vi "KH TURCK ETHERNETIP RFID Read.vi"(8 "error in":errorcluster, 11 "Response Data":T2={"ItemCount"=2, "AdressItem"={"TypeID"=0, "Length"=0, "Data"={"ConnectionIdentifier"=255, "SequenceNumber"=255}}, "DataItem"={"TypeID"=178, "Length"=8, "Data"=[], "Sequence Count"=8}} {"DataItem"."Data" format="%.0x"; "DataItem"."TypeID" format="%.0x"; "AdressItem"."Data"."ConnectionIdentifier" format="%.0x"; "AdressItem"."TypeID" format="%.0x"; "ItemCount" format="%.0x"}) -> (0 "error out":errorcluster, 3 "RFID_Read":T1[](array[typedef]))   [LabVIEW 2021]
uses:
  KH TURCK ETHERNETIP TDefCluster TBEN-S2-2RFID-4DXP Input Values.ctl
  KH EthernetIP 17.19/KH_EthernetIP_Globals.vi
  KH TURCK ETHERNETIP RFID Global.vi
  KH TURCK ETHERNETIP Global.vi
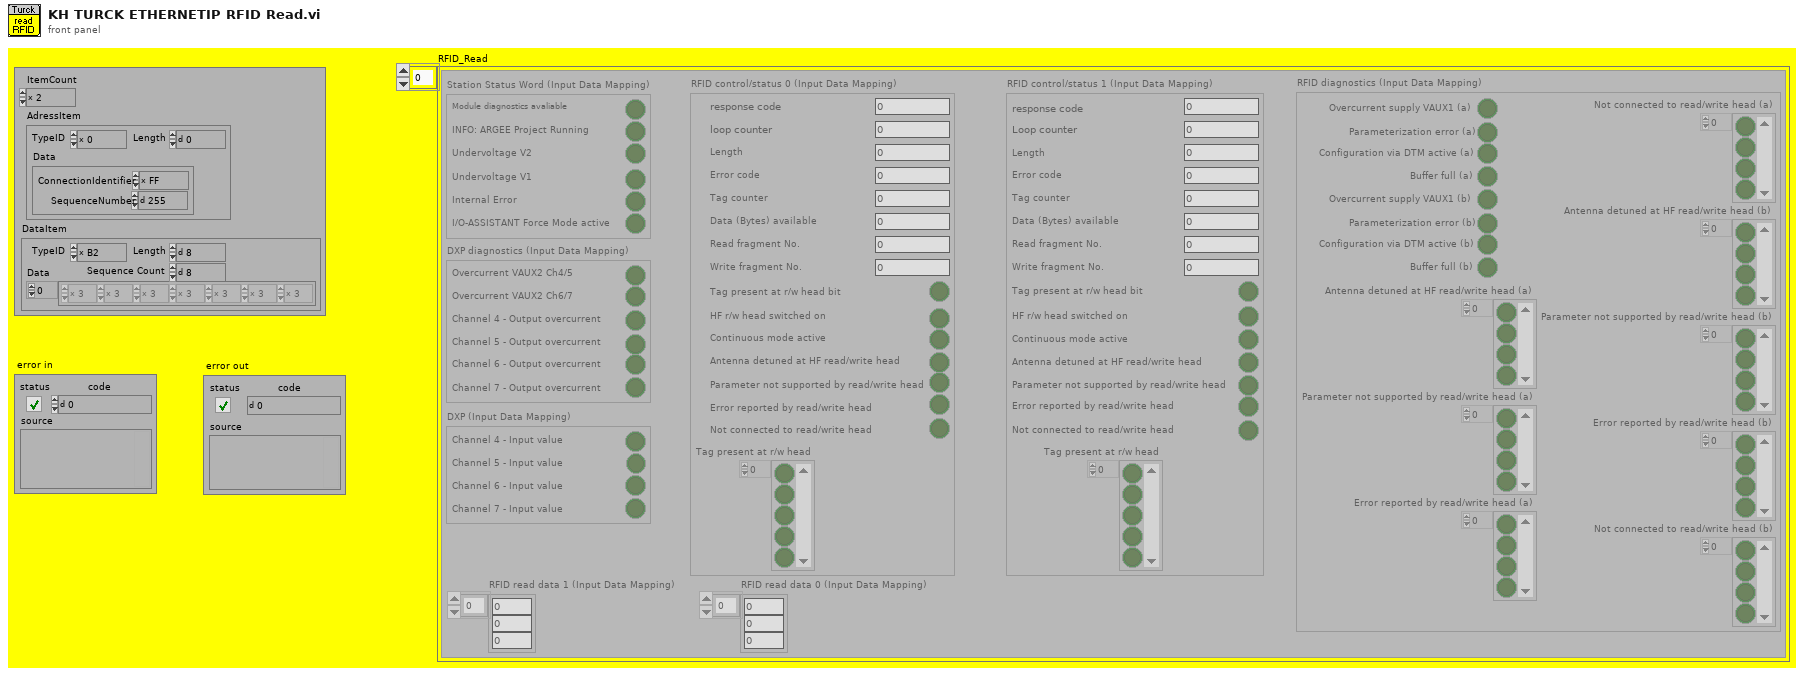
[diagram p1: front panel]
types:
  T1 = typedef "KH TURCK ETHERNETIP TDefCluster TBEN-S2-2RFID-4DXP Input Values.ctl" = cluster{"Station Status Word (Input Data Mapping)":cluster{"Module diagnostics avaliable":bool, "INFO: ARGEE Project Running":bool, "Undervoltage V2":bool, "Undervoltage V1":bool, "Internal Error":bool, "I/O-ASSISTANT Force Mode active":bool}, "RFID control/status 0 (Input Data Mapping)":cluster{"Tag present at r/w head":bool[], "response code":u16, "loop counter":u8, "Length":u16, "Error code":u16, "Tag counter":u16, "Data (Bytes) available":u16, "Read fragment No.":u8, "Write fragment No.":u8, "Tag present at r/w head bit":bool, "HF r/w head switched on":bool, "Continuous mode active":bool, "Antenna detuned at HF read/write head":bool, "Parameter not supported by read/write head":bool, "Error reported by read/write head":bool, "Not connected to read/write head":bool}, "RFID read data 0 (Input Data Mapping)":u8[], "RFID control/status 1 (Input Data Mapping)":cluster{"response code":u16, "Loop counter":u8, "Length":u16, "Error code":u16, "Tag counter":u16, "Data (Bytes) available":u16, "Read fragment No.":u8, "Write fragment No.":u8, "Tag present at r/w head bit":bool, "HF r/w head switched on":bool, "Continuous mode active":bool, "Antenna detuned at HF read/write head":bool, "Parameter not supported by read/write head":bool, "Error reported by read/write head":bool, "Not connected to read/write head":bool, "Tag present at r/w head":bool[]}, "RFID read data 1 (Input Data Mapping)":u8[], "RFID diagnostics (Input Data Mapping)":cluster{"Overcurrent supply VAUX1 (a)":bool, "Parameterization error (a)":bool, "Configuration via DTM active (a)":bool, "Buffer full (a)":bool, "Antenna detuned at HF read/write head (a)":bool[], "Parameter not supported by read/write head (a)":bool[], "Error reported by read/write head (a)":bool[], "Not connected to read/write head (a)":bool[], "Overcurrent supply VAUX1 (b)":bool, "Parameterization error (b)":bool, "Configuration via DTM active (b)":bool, "Buffer full (b)":bool, "Antenna detuned at HF read/write head (b)":bool[], "Parameter not supported by read/write head (b)":bool[], "Error reported by read/write head (b)":bool[], "Not connected to read/write head (b)":bool[]}, "DXP diagnostics (Input Data Mapping)":cluster{"Overcurrent VAUX2 Ch4/5":bool, "Overcurrent VAUX2 Ch6/7":bool, "Channel 4 - Output overcurrent":bool, "Channel 5 - Output overcurrent":bool, "Channel 6 - Output overcurrent":bool, "Channel 7 - Output overcurrent":bool}, "DXP (Input Data Mapping)":cluster{"Channel 4 - Input value":bool, "Channel 5 - Input value":bool, "Channel 6 - Input value":bool, "Channel 7 - Input value":bool}}
  T2 = cluster{"ItemCount":u16, "AdressItem":cluster{"TypeID":u16, "Length":u16, "Data":cluster{"ConnectionIdentifier":u32, "SequenceNumber":u32}}, "DataItem":cluster{"TypeID":u16, "Length":u16, "Data":u8[], "Sequence Count":u16}}
  T3 = typedef "KH EthernetIPConfig TDef Config.ctl" = cluster{"Typ":T4, "Name":string, "Nr.":i32, "InputOutput":enum16{"Input", "Output"}[]}
  T4 = typedef "KH EthernetIPConfig TypeDefs ModuleTyp.ctl" = enum16{"TBEN-S2-4AI", "TBEN-S1-8DXP", "TBEN-S2-2RFID-4DXP", "TBEN-S2-4AO", "TBEN-S2-4IOL"}
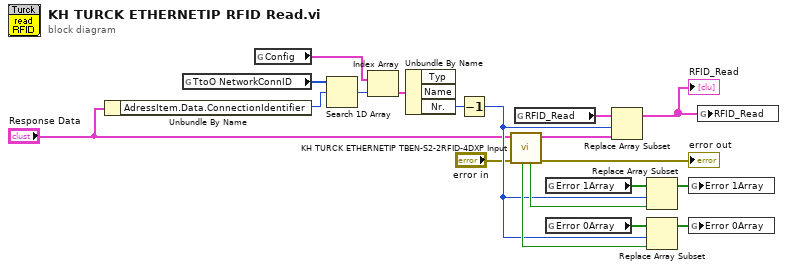
[diagram p0: block diagram]
diagram:
  n1 = Unbundle By Name("Response Data") -> ("AdressItem.Data.ConnectionIdentifier"=w19:u32)
  n2 = global read "KH_EthernetIP_Globals.vi" "TtoO NetworkConnID"() -> (w14:u32[])
  n3 = global read "KH_EthernetIP_Globals.vi" "Config"() -> (w15:T3[])
  n4 = Search 1D Array(1D array=w14, element=w19) -> (index of element=w18:i32)  [unwired: 1 in]
  n5 = Index Array(array=w15, index=w18) -> (element=w16:T3)
  n6 = Unbundle By Name(w16) -> ("Nr."=w17:i32)  [unwired: 2 out]
  n7 = Decrement(x=w17) -> (x-1=w6:i32)
  n8 = call "KH TURCK ETHERNETIP TBEN-S2-2RFID-4DXP Input.vi"("error in"="error in", "Response Data"="Response Data") -> ("error out"=→"error out":errorcluster, "Cluster"=w8:T1, "Error1"=w13:bool, "Error0"=w7:bool)  [unwired: 3 in, 3 out]
  n9 = global read "KH TURCK ETHERNETIP Global.vi" "RFID_Read"() -> (w2:T1[])
  n10 = global read "KH TURCK ETHERNETIP RFID Global.vi" "Error 1Array"() -> (w12:bool[])
  n11 = global read "KH TURCK ETHERNETIP RFID Global.vi" "Error 0Array"() -> (w9:bool[])
  n12 = Replace Array Subset(array=w2, new element=w8, index=w6) -> (w1:T1[])
  "RFID_Read" <- w1
  n13 = Replace Array Subset(array=w12, new element=w13, index=w6) -> (w11:bool[])
  n14 = Replace Array Subset(array=w9, new element=w7, index=w6) -> (w10:bool[])
  n15 = global write "KH TURCK ETHERNETIP RFID Global.vi" "Error 1Array"(w11) -> ()
  n16 = global write "KH TURCK ETHERNETIP RFID Global.vi" "Error 0Array"(w10) -> ()
  n17 = global write "KH TURCK ETHERNETIP Global.vi" "RFID_Read"(w1) -> ()
